vi "Handle Reply Msg.vi"(8 "error in (no error)":errorcluster, 9 "Panel Controller":refnum<class "Panel Controller Interface.lvclass">, 10 "EditPanel API in":refnum<class "EditPanel API.lvclass">, 11 "Console Reply Add Control.lvclass":refnum<class "Console Reply Add Control.lvclass">) -> (0 "error out":errorcluster, 2 "EditPanel API out":refnum<class "EditPanel API.lvclass">)   [LabVIEW 2015, in "Console Reply Add Control.lvclass"]
uses:
  Console Reply Add Control.lvclass
  _Depences/Panel API/EditPanel_class/EditPanel API.lvclass
  _Depences/Panel API/Panel Control_Interface/Panel_interface/Panel Controller Interface.lvclass
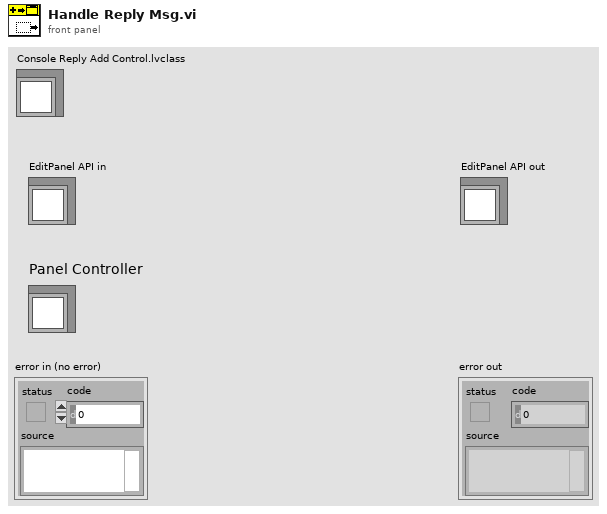
[diagram p1: front panel]
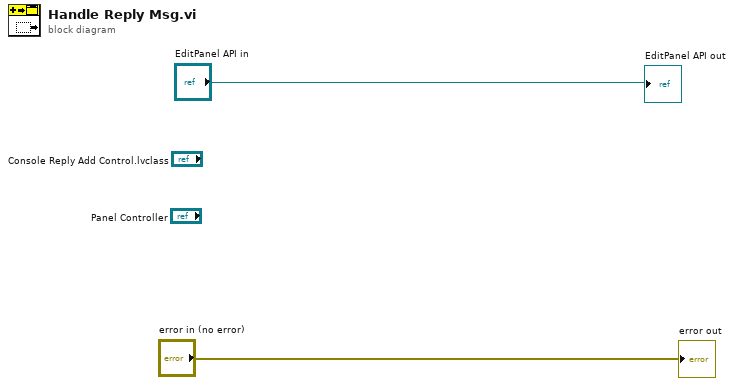
[diagram p0: block diagram]
diagram:
  "error out" <- "error in (no error)"
  "EditPanel API out" <- "EditPanel API in"
